vi "Write ID.vi"(8 "error in (no error)":errorcluster, 10 "ID":string, 11 "PID Loop in":refnum<class "PID Loop.lvclass">) -> (0 "error out":errorcluster, 3 "PID Loop out":refnum<class "PID Loop.lvclass">)   [LabVIEW 2014, in "PID Loop.lvclass"]
uses:
  PID Loop.lvclass
  PID Loop.lvclass/PID Loop.ctl
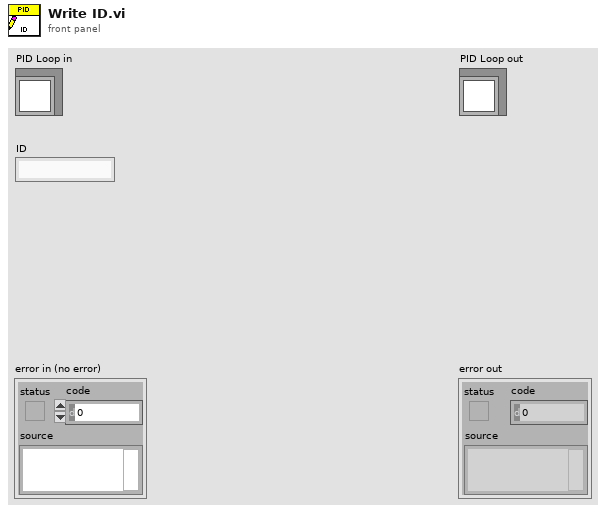
[diagram p1: front panel]
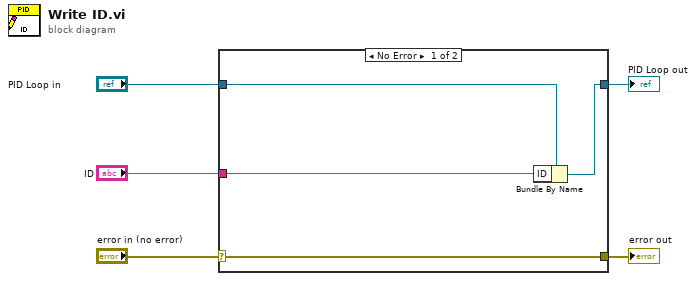
[diagram p0: block diagram]
diagram:
  n1 = case shown="No Error" "error in (no error)" {
    selector: "error in (no error)" -> [w9 w10]
    tunnel: [w9 w10] -> w4
    tunnel: [w7 w11] -> w2
    tunnel: "PID Loop in" -> [w8 w11]
    tunnel: "ID" -> [w6 _]
    frame No Error {
      n2 = Bundle By Name(cluster=w8, "ID"=w6) -> (w7:refnum<class "PID Loop.lvclass">)
    }
    frame Error {
    }
  }
  "error out" <- w4
  "PID Loop out" <- w2
